vi "GetParam.vi"(8 "error in (no error)":errorcluster caption="entrée d'erreur (pas d'erreur)", 11 "KNNImputer.lvclass":refnum<class "KNNImputer.lvclass">) -> (0 "error out":errorcluster caption="sortie d'erreur", 2 "KNNImputer":T1={"missing_values"="nan", "n_neighbors"=5, "weights"="uniform", "metric"="nan_euclidean", "copy"=TRUE, "add_indicator"=FALSE}, 3 "KNNImputer.lvclass":refnum<class "KNNImputer.lvclass">)   [LabVIEW 2020, in "KNNImputer.lvclass"]
doc: "Get Parameters"
uses:
  KNNImputer.lvclass
  KNNImputer.lvclass/KNNImputer.ctl
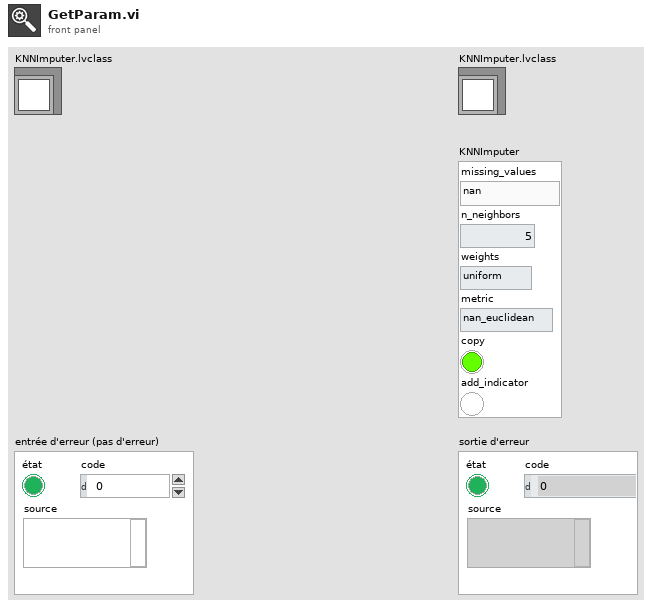
[diagram p1: front panel]
types:
  T1 = cluster{"missing_values":string, "n_neighbors":i32, "weights":string, "metric":string, "copy":bool, "add_indicator":bool}
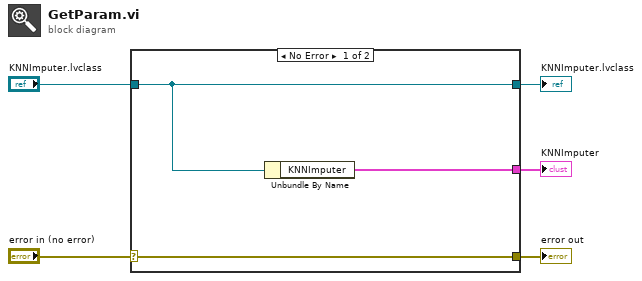
[diagram p0: block diagram]
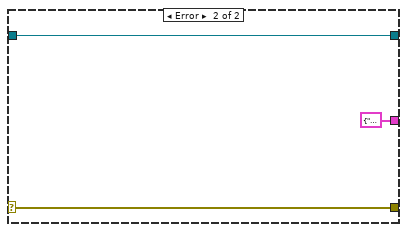
[diagram p2: hidden frame]
diagram:
  n1 = case shown="No Error" "error in (no error)" {
    selector: "error in (no error)" -> [w8 w10]
    tunnel: [w8 w10] -> w4
    tunnel: [w7 w11] -> w2
    tunnel: "KNNImputer.lvclass" -> [w7 w11]
    tunnel: [w6 T1 {"missing_values"="", "n_neighbors"=0, "weights"="", "metric"="", "copy"=FALSE, "add_indicator"=FALSE} ("KNNImputer")] -> w1
    frame No Error {
      n2 = Unbundle By Name(w7) -> ("KNNImputer"=w6:T1)
    }
    frame Error {
    }
  }
  "error out" <- w4
  "KNNImputer.lvclass" <- w2
  "KNNImputer" <- w1
